vi "DC Source Core Logic.vi"(8 "error in":errorcluster, 9 "measurement configuration":T1, 10 "instrument handle":refnum<k15>, 11 "channel list":string) -> (0 "error out":errorcluster, 1 "calculated power":dbl, 2 "measured current":dbl, 3 "instrument handle out":refnum<k15>, 4 "in compliance?":bool, 5 "measured voltage":dbl)   [LabVIEW 2024, in "NIDCPowerSupplyAndSource.lvlib"]
uses:
  NIDCPowerSupplyAndSource.lvlib
  Measurement Configuration.ctl
  <instrlib>/niDCPower/nidcpower.llb/niDCPower Source Mode.ctl
  <instrlib>/niDCPower/nidcpower.llb/niDCPower Output Function.ctl
  <instrlib>/niDCPower/nidcpower.llb/niDCPower Wait For Event - Event.ctl
  <instrlib>/niDCPower/nidcpower.llb/niDCPower Measurement Type.ctl
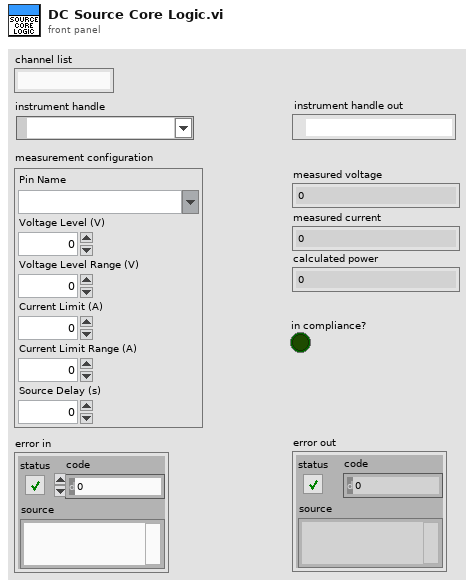
[diagram p1: front panel]
types:
  T1 = typedef "NIDCPowerSupplyAndSource.lvlib/Measurement Configuration.ctl" = cluster{"Pin Name":string, "Voltage Level (V)":dbl, "Voltage Level Range (V)":dbl, "Current Limit (A)":dbl, "Current Limit Range (A)":dbl, "Source Delay (s)":dbl}
  T2 = typedef "niDCPower Measurement Type.ctl" = i32
  T3 = typedef "niDCPower Wait For Event - Event.ctl" = i32
  T4 = typedef "niDCPower Output Function.ctl" = i32
  T5 = typedef "niDCPower Source Mode.ctl" = i32
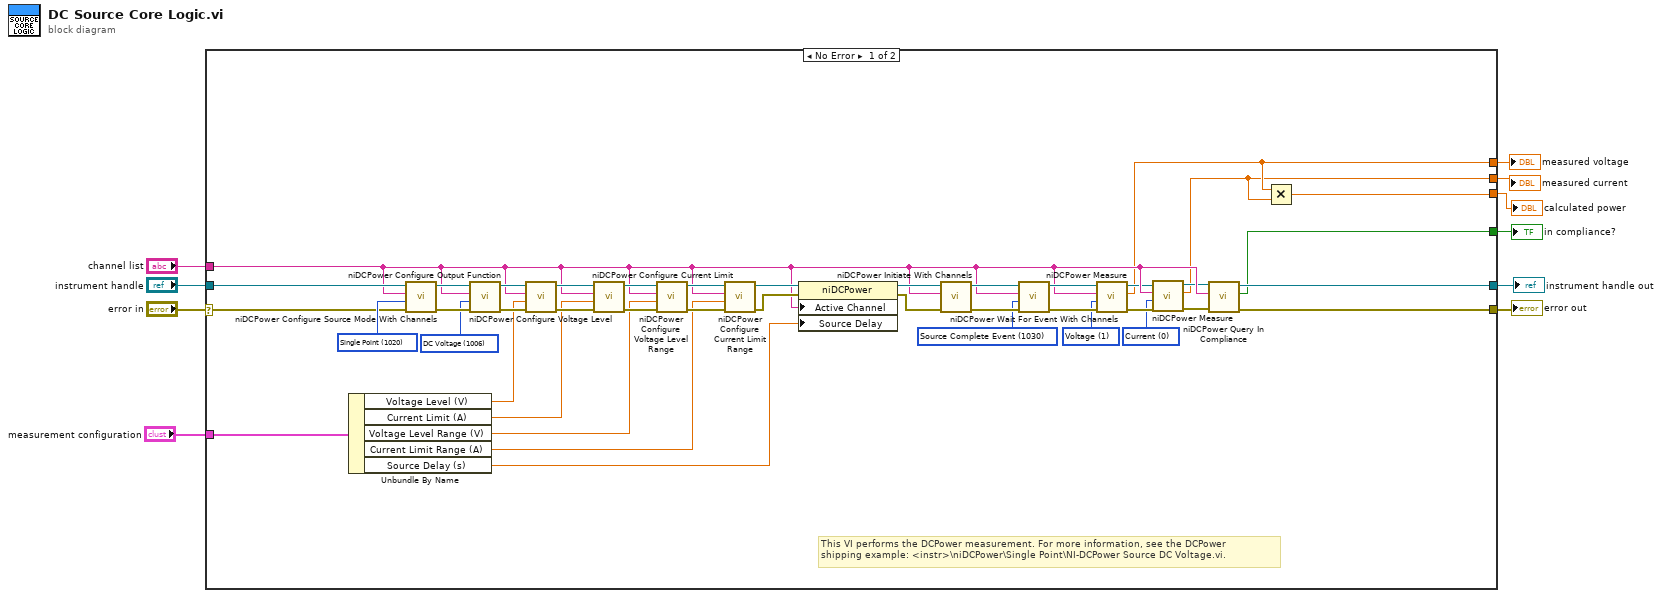
[diagram p0: block diagram]
diagram:
  n1 = case shown="No Error" "error in" {
    selector: "error in" -> [w27 w53]
    tunnel: [w24 w53] -> w10
    tunnel: "instrument handle" -> [w28 w54]
    tunnel: [w25 w54] -> w8
    tunnel: "channel list" -> [w21 _]
    tunnel: "measurement configuration" -> [w26 _]
    tunnel: [w14 _] -> w4
    tunnel: [w13 _] -> w3
    tunnel: [w12 _] -> w2
    tunnel: [w11 _] -> w1
    frame No Error {
      w15 = T2 0 items=["Current", "Voltage"] ("measurement type")
      w16 = T2 1 items=["Current", "Voltage"] ("measurement type")
      w32 = T3 1030 items=["Source Complete Event"=1030, "Measure Complete Event"=1031, "Sequence Iteration Complete Event"=1032, "Sequence Engine Done Event"=1033, "Pulse Complete Event"=1051, "Ready For Pulse Trigger Event"=1052] ("event")
      w35 = T4 1006 items=["DC Voltage"=1006, "DC Current"=1007, "Pulse Voltage"=1049, "Pulse Current"=1050] ("output function")
      w36 = T5 1020 items=["Single Point"=1020, "Sequence"=1021] ("source mode")
      # "This VI performs the DCPower measurement. For more information, see the DCPower\nshipping example: <instr>\\niDCPower\\Single Point\\NI-DCPower Source DC Voltage.vi."
      n2 = Unbundle By Name(w26) -> ("Voltage Level (V)"=w34:dbl, "Current Limit (A)"=w33:dbl, "Voltage Level Range (V)"=w31:dbl, "Current Limit Range (A)"=w30:dbl, "Source Delay (s)"=w29:dbl)
      n3 = call <instrlib>:"niDCPower Configure Source Mode With Channels.vi"("error in (no error)"=w27, "source mode"=w36, "channel name"=w21, "instrument handle"=w28) -> ("error out"=w50:errorcluster, "instrument handle out"=w49:refnum<k15>)  [unwired: 6 in]
      n4 = call <instrlib>:"niDCPower Configure Output Function.vi"("error in (no error)"=w50, "output function"=w35, "channel name"=w21, "instrument handle"=w49) -> ("error out"=w37:errorcluster, "instrument handle out"=w38:refnum<k15>)  [unwired: 6 out]
      n5 = call <instrlib>:"niDCPower Configure Voltage Level.vi"("error in (no error)"=w37, "voltage level"=w34, "channel name"=w21, "instrument handle"=w38) -> ("error out"=w51:errorcluster, "instrument handle out"=w52:refnum<k15>)  [unwired: 6 out]
      n6 = call <instrlib>:"niDCPower Configure Current Limit.vi"("error in (no error)"=w51, "current limit"=w33, "channel name"=w21, "instrument handle"=w52) -> ("error out"=w48:errorcluster, "instrument handle out"=w47:refnum<k15>)  [unwired: 1 in, 5 out]
      n7 = call <instrlib>:"niDCPower Configure Voltage Level Range.vi"("error in (no error)"=w48, "voltage level range"=w31, "channel name"=w21, "instrument handle"=w47) -> ("error out"=w46:errorcluster, "instrument handle out"=w45:refnum<k15>)  [unwired: 6 out]
      n8 = call <instrlib>:"niDCPower Configure Current Limit Range.vi"("error in (no error)"=w46, "current limit range"=w30, "channel name"=w21, "instrument handle"=w45) -> ("error out"=w41:errorcluster, "instrument handle out"=w44:refnum<k15>)  [unwired: 6 out]
      n9 = property class="niDCPower"(reference=w44, error in=w41, "Active Channel"=w21, "Source Delay"=w29) -> (reference out=w43:refnum<k15>, error out=w42:errorcluster)
      n10 = call <instrlib>:"niDCPower Initiate With Channels.vi"("error in (no error)"=w42, "channel name"=w21, "instrument handle"=w43) -> ("error out"=w39:errorcluster, "instrument handle out"=w40:refnum<k15>)  [unwired: 7 in]
      n11 = call <instrlib>:"niDCPower Wait For Event With Channels.vi"("error in (no error)"=w39, "event"=w32, "channel name"=w21, "instrument handle"=w40) -> ("error out"=w22:errorcluster, "instrument handle out"=w23:refnum<k15>)  [unwired: 6 in]
      n12 = call <instrlib>:"niDCPower Measure.vi"("error in (no error)"=w22, "measurement type"=w16, "channel name"=w21, "instrument handle"=w23) -> ("error out"=w18:errorcluster, "measurement"=w14:dbl, "instrument handle out"=w20:refnum<k15>)  [unwired: 5 in]
      n13 = call <instrlib>:"niDCPower Measure.vi"("error in (no error)"=w18, "measurement type"=w15, "channel name"=w21, "instrument handle"=w20) -> ("error out"=w17:errorcluster, "measurement"=w13:dbl, "instrument handle out"=w19:refnum<k15>)  [unwired: 5 in]
      n14 = call <instrlib>:"niDCPower Query In Compliance.vi"("error in (no error)"=w17, "channel name"=w21, "instrument handle"=w19) -> ("error out"=w24:errorcluster, "in compliance?"=w11:bool, "instrument handle out"=w25:refnum<k15>)  [unwired: 6 out]
      n15 = Multiply(x=w14, y=w13) -> (x*y=w12:dbl)
    }
    frame Error {
    }
  }
  "error out" <- w10
  "instrument handle out" <- w8
  "measured voltage" <- w4
  "measured current" <- w3
  "calculated power" <- w2
  "in compliance?" <- w1
